vi "Get Count.vi"(10 "Fit Array":i32[](array[numeric]), 11 "Stream Array":T1[](array[typedef])) -> (3 "Count Out":u64)   [LabVIEW 2023]
uses:
  ENUM_Type.ctl
  Cluster Array Key.ctl
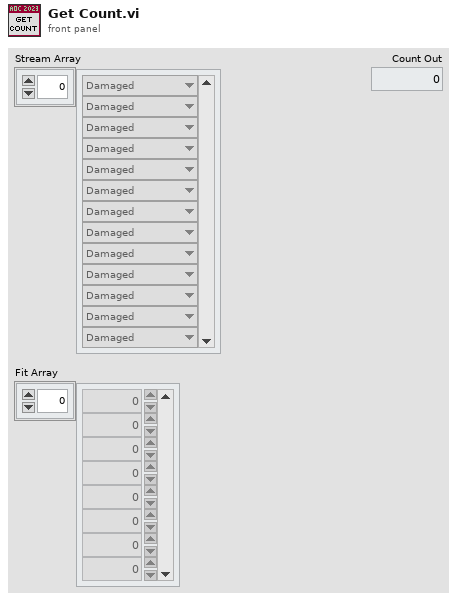
[diagram p1: front panel]
types:
  T1 = typedef "ENUM_Type.ctl" = enum16{"Damaged", "Operational", "Unknown"}
  T2 = typedef "Cluster Array Key.ctl" = cluster{"Streams":T1[], "Fits":i32[]}
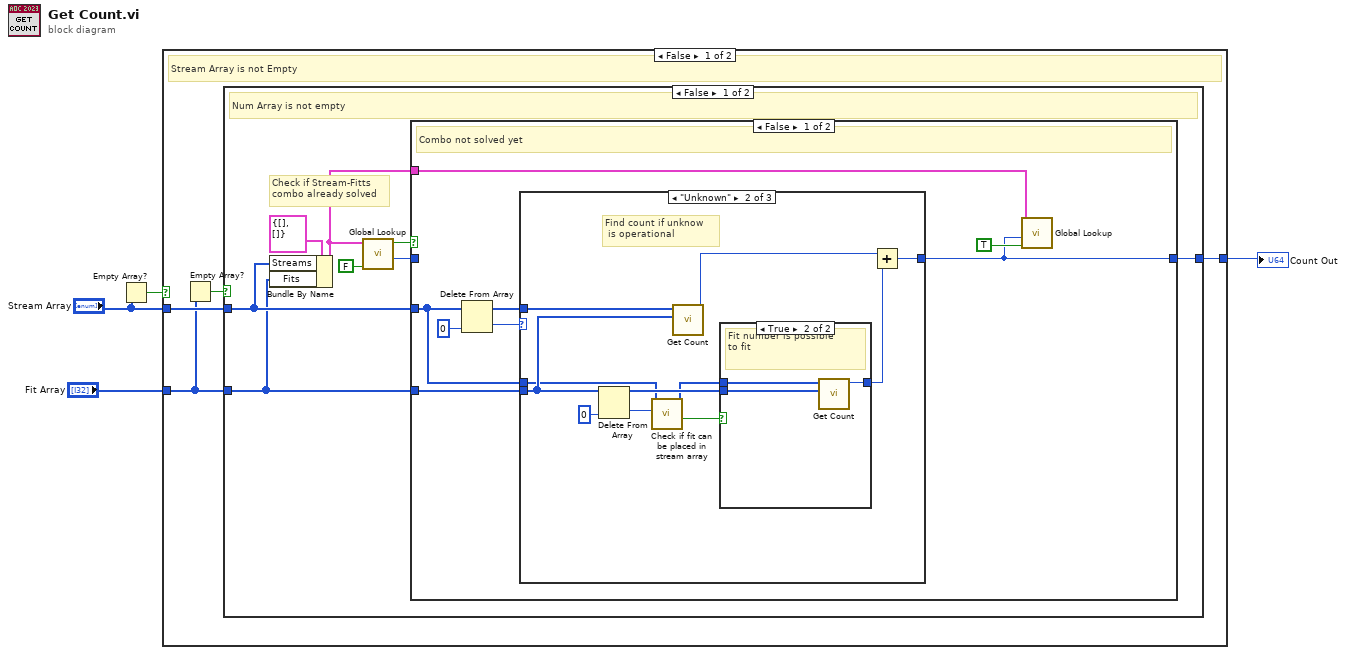
[diagram p0: block diagram]
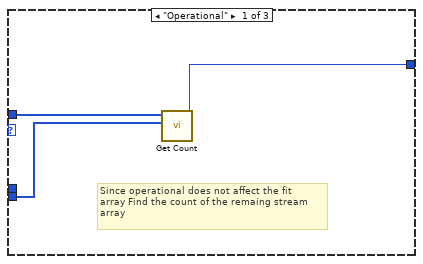
[diagram p2: hidden frame]
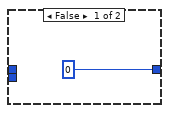
[diagram p3: hidden frame]
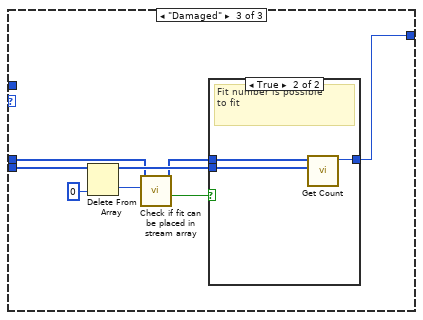
[diagram p4: hidden frame]
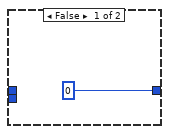
[diagram p5: hidden frame]
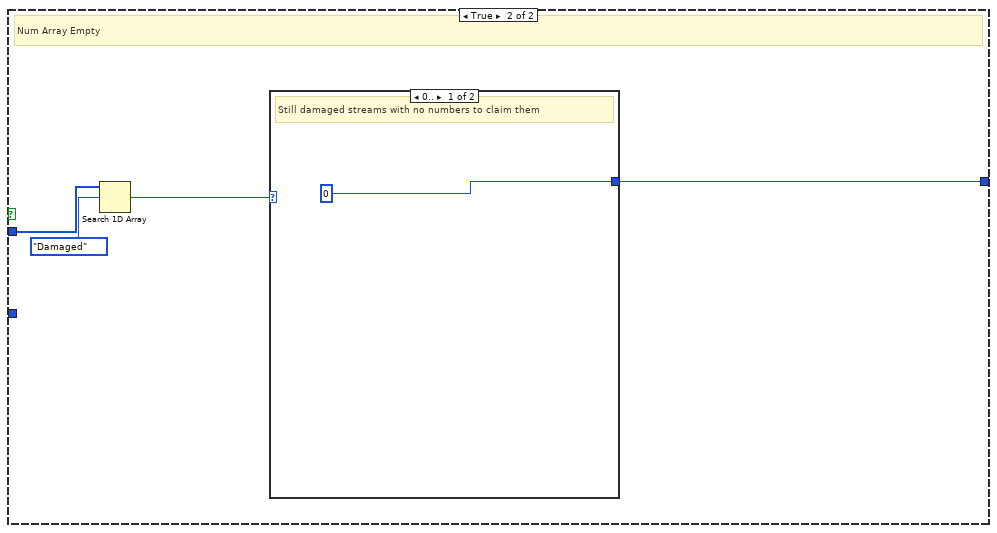
[diagram p7: hidden frame]
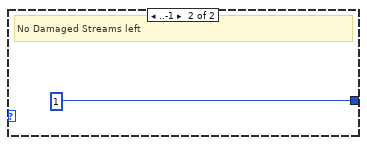
[diagram p8: hidden frame]
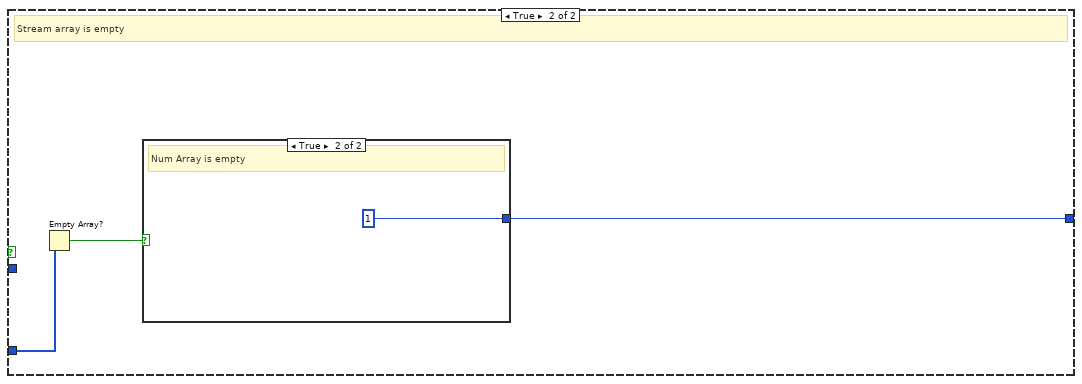
[diagram p9: hidden frame]
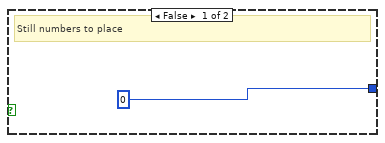
[diagram p10: hidden frame]
diagram:
  n1 = Empty Array?(array="Stream Array") -> (empty?=w3:bool)
  n2 = case shown="False" w3 {
    tunnel: "Fit Array" -> [w7 w64]
    tunnel: "Stream Array" -> [w8 _]
    tunnel: [w5 w62] -> w1
    frame False {
      # "Stream Array is not Empty"
      n3 = Empty Array?(array=w7) -> (empty?=w6:bool)
      n4 = case shown="False" w6 {
        tunnel: w8 -> [w12 w59]
        tunnel: w7 -> [w11 _]
        tunnel: [w10 w56] -> w5
        frame False {
          # "Check if Stream-Fitts\ncombo already solved"
          # "Num Array is not empty"
          n5 = Bundle By Name(cluster=T2 {"Streams"=[], "Fits"=[]} ("Key"), "Streams"=w12, "Fits"=w11) -> (w9:T2)
          n6 = call "Global Lookup.vi"("Read(f) Write(T)"=FALSE, "Key"=w9) -> ("Value Out"=w13:u64, "Key Found Out"=w14:bool)  [unwired: 8 in]
          n7 = case shown="False" w14 {
            tunnel: [w17 w55] -> w10
            tunnel: w13 -> [_ w55]
            tunnel: w12 -> [w20 _]
            tunnel: w11 -> [w21 _]
            tunnel: w9 -> [w18 _]
            frame False {
              # "Combo not solved yet"
              n8 = Delete From Array(array=w20, index=0) -> (deleted portion=w24:T1, array with subset deleted=w22:T1[])  [unwired: 1 in]
              n9 = case shown="\"Unknown\"" w24 {
                tunnel: w22 -> [w27 w35 _]
                tunnel: w21 -> [w26 w32 w48]
                tunnel: [w25 w37 w43] -> w17
                tunnel: w20 -> [_ w30 w46]
                frame "Operational" {
                  # "Since operational does not affect the fit\narray Find the count of the remaing stream\narray"
                  n10 = call "Get Count.vi"("Fit Array"=w26, "Stream Array"=w27) -> ("Count Out"=w25:u64)  [unwired: 9 in]
                }
                frame "Unknown" {
                  # "Find count if unknow\n is operational"
                  n11 = Delete From Array(array=w32, index=0) -> (deleted portion=w28:i32, array with subset deleted=w33:i32[])  [unwired: 1 in]
                  n12 = call "Check if fit can be placed in stream array.vi"("Fit Number"=w28, "Stream Array"=w30) -> ("Possible Out"=w29:bool, "Remaining Stream Out"=w31:T1[])  [unwired: 8 in]
                  n13 = call "Get Count.vi"("Fit Array"=w32, "Stream Array"=w35) -> ("Count Out"=w38:u64)  [unwired: 9 in]
                  n14 = case shown="True" w29 {
                    tunnel: [0 ("Count Out") w42] -> w36
                    tunnel: w31 -> [_ w41]
                    tunnel: w33 -> [_ w40]
                    frame False {
                    }
                    frame True {
                      # "Fit number is possible\nto fit"
                      n15 = call "Get Count.vi"("Fit Array"=w40, "Stream Array"=w41) -> ("Count Out"=w42:u64)  [unwired: 9 in]
                    }
                  }
                  n16 = Add(x=w38, y=w36) -> (x+y=w37:u64)
                }
                frame "Damaged" {
                  n17 = Delete From Array(array=w48, index=0) -> (deleted portion=w44:i32, array with subset deleted=w49:i32[])  [unwired: 1 in]
                  n18 = call "Check if fit can be placed in stream array.vi"("Fit Number"=w44, "Stream Array"=w46) -> ("Possible Out"=w45:bool, "Remaining Stream Out"=w47:T1[])  [unwired: 8 in]
                  n19 = case shown="True" w45 {
                    tunnel: [0 ("Count Out") w54] -> w43
                    tunnel: w47 -> [_ w53]
                    tunnel: w49 -> [_ w52]
                    frame False {
                    }
                    frame True {
                      # "Fit number is possible\nto fit"
                      n20 = call "Get Count.vi"("Fit Array"=w52, "Stream Array"=w53) -> ("Count Out"=w54:u64)  [unwired: 9 in]
                    }
                  }
                }
              }
              n21 = call "Global Lookup.vi"("Read(f) Write(T)"=TRUE, "Value"=w17, "Key"=w18) -> ()  [unwired: 7 in, 2 out]
            }
            frame True {
              # "Combo already solved for use previous number"
            }
          }
        }
        frame True {
          # "Num Array Empty"
          n22 = Search 1D Array(1D array=w59, element=ENUM_Type."Damaged") -> (index of element=w57:i32)  [unwired: 1 in]
          n23 = case shown="0.." w57 {
            tunnel: [u64 0 u64 1] -> w56
            frame 0.. {
              # "Still damaged streams with no numbers to claim them"
            }
            frame ..-1 {
              # "No Damaged Streams left"
            }
          }
        }
      }
    }
    frame True {
      # "Stream array is empty"
      n24 = Empty Array?(array=w64) -> (empty?=w63:bool)
      n25 = case shown="True" w63 {
        tunnel: [u64 0 u64 1] -> w62
        frame False {
          # "Still numbers to place"
        }
        frame True {
          # "Num Array is empty"
        }
      }
    }
  }
  "Count Out" <- w1
